vi "Get Port Number.vi"(0 "LV DEV.lvclass":refnum<class "LV DEV.lvclass">, 11 "Error In":errorcluster) -> (4 "LV DEV.lvclass":refnum<class "LV DEV.lvclass">, 6 "Machine name":string, 8 "Port Number":u16, 15 "error Out":errorcluster)   [LabVIEW 2019, in "LV DEV.lvclass"]
uses:
  LV DEV.lvclass
  LV DEV.lvclass/LV DEV.ctl
  property/Read LabVIEW version.vi
  <vilib>/Utility/config.llb/Read Key (U32).vi
  <vilib>/Utility/config.llb/NI_LVConfig.lvlib
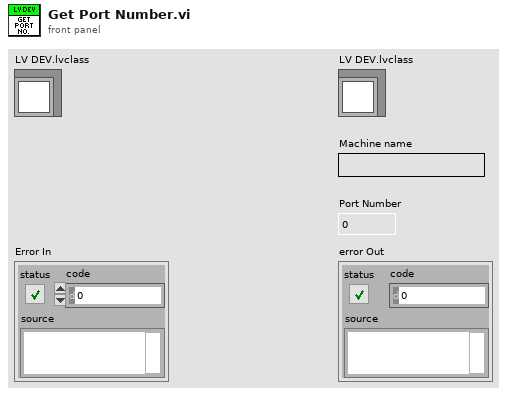
[diagram p1: front panel]
types:
  T1 = typedef "NI_LVConfig.lvlib/Config Data RefNum.ctl" = refnum<k1>
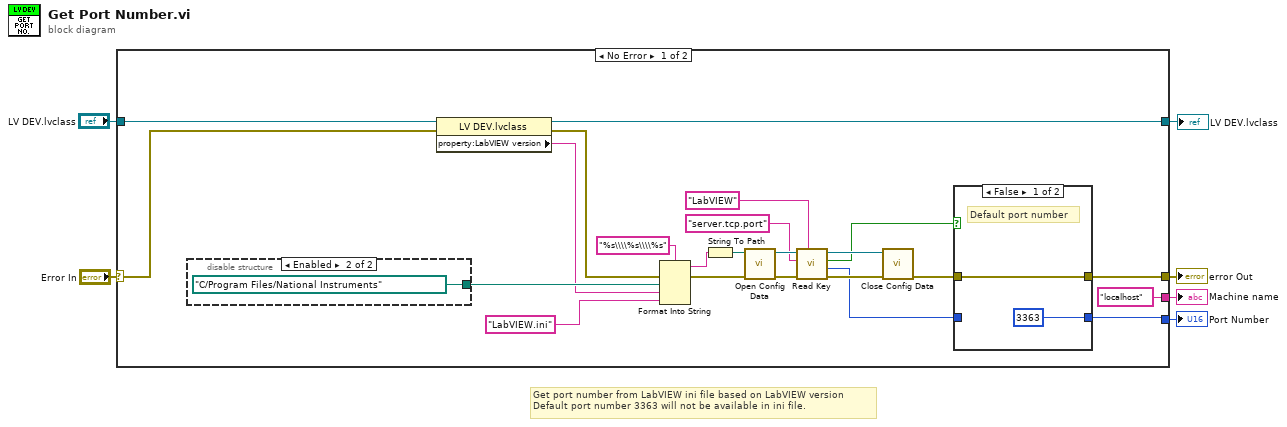
[diagram p0: block diagram]
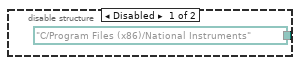
[diagram p2: hidden frame]
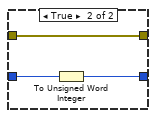
[diagram p3: hidden frame]
diagram:
  # "Get port number from LabVIEW ini file based on LabVIEW version\nDefault port number 3363 will not be available in ini file."
  n1 = case shown="No Error" "Error In" {
    selector: "Error In" -> [w26 w38]
    tunnel: [w10 w38] -> w5
    tunnel: "LV DEV.lvclass" -> [w28 w37]
    tunnel: [w27 w37] -> w1
    tunnel: ["localhost" _] -> w4
    tunnel: [w7 _] -> w3
    frame No Error {
      n2 = disable-structure shown="Enabled" {
        disable-tunnel: [path "C:/Program Files (x86)/National Instruments" path "C:/Program Files/National Instruments"] -> w24
        frame Disabled {
        }
        frame Enabled {
        }
      }
      n3 = property class="LV DEV.lvclass"(reference=w28, error in=w26) -> (reference out=w27:refnum<class "LV DEV.lvclass">, error out=w25:errorcluster, "property:LabVIEW version"=w23:string)
      n4 = Format Into String(format string="%s\\\\%s\\\\%s", error in=w25, w24, w23, "LabVIEW.ini" ("input 3")) -> (resulting string=w20:string, error out=w19:errorcluster)  [unwired: 1 in]
      n5 = String To Path(string=w20) -> (path=w18:path)
      n6 = call <vilib>:"Open Config Data.vi"("error in (no error)"=w19, "configuration file path"=w18) -> ("error out"=w17:errorcluster, "refnum"=w15:T1)  [unwired: 7 in, 1 out]
      n7 = call-poly <vilib>:"Read Key.vi"("section"="LabVIEW", "error in (no error)"=w17, "key"="server.tcp.port", "refnum"=w15) -> ("error out"=w16:errorcluster, "value"=w8:u32, "found?"=w9:bool, "refnum out"=w13:T1)  [unwired: 4 in]
      n8 = call <vilib>:"Close Config Data.vi"("error in (no error)"=w16, "refnum"=w13) -> ("error out"=w11:errorcluster)  [unwired: 8 in, 1 out]
      n9 = case shown="False" w9 {
        tunnel: w11 -> [w33 w36]
        tunnel: [w33 w36] -> w10
        tunnel: [u16 3363 ("value") w34] -> w7
        tunnel: w8 -> [_ w35]
        frame False {
          # "Default port number"
        }
        frame True {
          n10 = To Unsigned Word Integer(number=w35) -> (unsigned 16bit integer=w34:u16)
        }
      }
    }
    frame Error {
    }
  }
  "error Out" <- w5
  "Port Number" <- w3
  "Machine name" <- w4
  "LV DEV.lvclass" <- w1
